vi "EMSA SpectralBandAcrossSegments.vi"(7 "sweeps":T1[](array[typedef])=[{"start"=30000.0, "stop"=300000.0, "bandwidth"=9000.0}, {"start"=300000.0, "stop"=3000000.0, "bandwidth"=9000.0}, {"start"=3000000.0, "stop"=30000000.0, "bandwidth"=9000.0}, {"start"=30000000.0, "stop"=100000000.0, "bandwidth"=120000.0}], 9 "stop frequency":dbl=-1.0, 10 "start frequency":dbl=-1.0, 11 "sweep in":cluster{"frequency":dbl[], "amplitude":dbl[]}={"frequency"=array[8000 elements], "amplitude"=array[8000 elements]}) -> (0 "stop index":i32, 1 "start index":i32, 3 "power in band":dbl)   [LabVIEW 2017, in "EmsaAnalysis.lvlib"]
uses:
  <vilib>/addons/InsightCM/Devices/Shared/Emsa/EmsaAnalysis/EmsaAnalysis.lvlib
  <vilib>/addons/InsightCM/Devices/Shared/Emsa/EmsaAnalysis/controls/sweepInfo.ctl
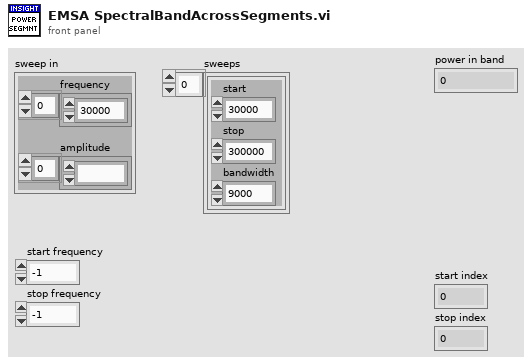
[diagram p1: front panel]
types:
  T1 = typedef "EmsaAnalysis.lvlib/sweepInfo.ctl" = cluster{"start":dbl, "stop":dbl, "bandwidth":dbl}
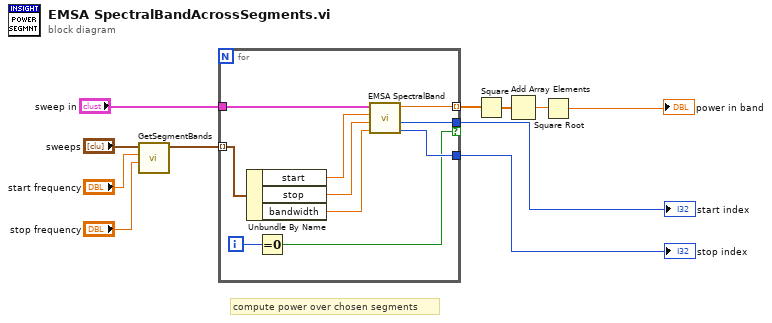
[diagram p0: block diagram]
diagram:
  # "compute power over chosen segments"
  n1 = call <vilib>:"GetSegmentBands.vi"("stop frequency"="stop frequency", "start frequency"="start frequency", "sweeps in"="sweeps") -> ("sweeps out"=w2:T1[])  [unwired: 8 in]
  n2 = for {
    tunnel: w2 -> [w21] mode=indexing
    tunnel: "sweep in" -> [w20]
    tunnel: [w16] -> w7 mode=indexing
    tunnel: [w15] -> w4 if=w12
    tunnel: [w14] -> w3
    i -> [w13]
    n3 = Unbundle By Name(w21) -> ("start"=w19:dbl, "stop"=w18:dbl, "bandwidth"=w17:dbl)
    n4 = Equal To 0?(x=w13) -> (x = 0?=w12:bool)
    n5 = call <vilib>:"EMSA SpectralBand.vi"("bandwidth"=w17, "stop frequency"=w18, "start frequency"=w19, "sweep in"=w20) -> ("stop index"=w14:i32, "start index"=w15:i32, "power in band"=w16:dbl)  [unwired: 5 in]
  }
  "start index" <- w4
  "stop index" <- w3
  n6 = Square(x=w7) -> (x^2=w8:dbl[])
  n7 = Add Array Elements(numeric array=w8) -> (sum=w6:dbl)
  n8 = Square Root(x=w6) -> (sqrt(x)=→"power in band":dbl)
